vi "XDimension Enum to String.vi"(11 "XDimension Enum":T1=enum."Time [sec]" caption="Value") -> (3 "element":string)   [LabVIEW 2017, in "GetSetShared.lvlib"]
uses:
  <vilib>/express/express signal manip/GetorSetDDTAttributes/Shared VIs/GetSetShared.lvlib
  <vilib>/express/express signal manip/GetorSetDDTAttributes/Shared VIs/XDimension.ctl
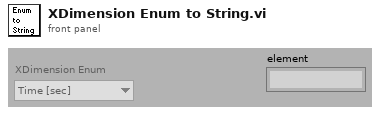
[diagram p1: front panel]
types:
  T1 = typedef "GetSetShared.lvlib/XDimension.ctl" = enum16{"No Unit [-]", "Time [sec]", "Frequency [Hz]"}
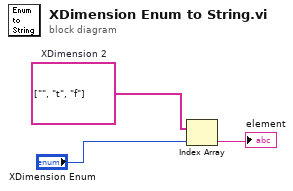
[diagram p0: block diagram]
diagram:
  w3 = string[] ["", "t", "f"]  # XDimension 2
  n1 = Index Array(array=w3, index="XDimension Enum") -> (element=→"element":string)
